vi "WILT Step 4.vi"(0 "Dryer Step 4 In":T8 {"Night Cycle Count" format="%04d"; "Day Cycle Count" format="%04d"}, 1 "Day/Night Cycle":T2, 2 "Step 3 Input":T6, 5 "Error In":errorcluster, 6 "Valve Status":T4, 7 "Agilent Valve and Switch Locations":T3[](array[typedef])=[{"Channel"="301", "Station"="1", "Label"="Water Valve", "Agilent Station"="2", "Data"=0.0}, {"Channel"="302", "Station"="2", "Label"="Water Valve", "Agilent Station"="2", "Data"=0.0}, {"Channel"="303", "Station"="3", "Label"="Water Valve", "Agilent Station"="2", "Data"=0.0}, {"Channel"="304", "Station"="4", "Label"="Water Valve", "Agilent Station"="2", "Data"=0.0}, {"Channel"="305", "Station"="5", "Label"="Water Valve", "Agilent Station"="2", "Data"=0.0}, {"Channel"="306", "Station"="6", "Label"="Water Valve", "Agilent Station"="2", "Data"=0.0}, {"Channel"="307", "Station"="7", "Label"="Water Valve", "Agilent Station"="2", "Data"=0.0}, {"Channel"="308", "Station"="8", "Label"="Water Valve", "Agilent Station"="2", "Data"=0.0}, {"Channel"="309", "Station"="9", "Label"="Water Valve", "Agilent Station"="2", "Data"=0.0}, {"Channel"="310", "Station"="10", "Label"="Water Valve", "Agilent Station"="2", "Data"=0.0}, {"Channel"="311", "Station"="11", "Label"="Water Valve", "Agilent Station"="2", "Data"=0.0}, {"Channel"="312", "Station"="12", "Label"="Water Valve", "Agilent Station"="2", "Data"=0.0}, {"Channel"="313", "Station"="13", "Label"="Water Valve", "Agilent Station"="2", "Data"=0.0}, {"Channel"="314", "Station"="14", "Label"="Water Valve", "Agilent Station"="2", "Data"=0.0}, {"Channel"="315", "Station"="15", "Label"="Water Valve", "Agilent Station"="2", "Data"=0.0}, {"Channel"="316", "Station"="16", "Label"="Water Valve", "Agilent Station"="2", "Data"=0.0}, {"Channel"="317", "Station"="17", "Label"="Water Valve", "Agilent Station"="2", "Data"=0.0}, {"Channel"="318", "Station"="18", "Label"="Water Valve", "Agilent Station"="2", "Data"=0.0}, {"Channel"="319", "Station"="19", "Label"="Water Valve", "Agilent Station"="2", "Data"=0.0}, {"Channel"="320", "Station"="20", "Label"="Water Valve", "Agilent Station"="2", "Data"=0.0}, {"Channel"="101", "Station"="21", "Label"="Water Valve", "Agilent Station"="3", "Data"=0.0}, {"Channel"="102", "Station"="22", "Label"="Water Valve", "Agilent Station"="3", "Data"=0.0}, {"Channel"="103", "Station"="23", "Label"="Water Valve", "Agilent Station"="3", "Data"=0.0}, {"Channel"="104", "Station"="24", "Label"="Water Valve", "Agilent Station"="3", "Data"=0.0}, {"Channel"="105", "Station"="25", "Label"="Water Valve", "Agilent Station"="3", "Data"=0.0}, {"Channel"="106", "Station"="26", "Label"="Water Valve", "Agilent Station"="3", "Data"=0.0}, {"Channel"="107", "Station"="27", "Label"="Water Valve", "Agilent Station"="3", "Data"=0.0}, {"Channel"="108", "Station"="28", "Label"="Water Valve", "Agilent Station"="3", "Data"=0.0}, {"Channel"="109", "Station"="29", "Label"="Water Valve", "Agilent Station"="3", "Data"=0.0}, {"Channel"="110", "Station"="30", "Label"="Water Valve", "Agilent Station"="3", "Data"=0.0}, {"Channel"="111", "Station"="31", "Label"="Water Valve", "Agilent Station"="3", "Data"=0.0}, {"Channel"="112", "Station"="32", "Label"="Water Valve", "Agilent Station"="3", "Data"=0.0}, {"Channel"="101", "Station"="33", "Label"="Water Valve", "Agilent Station"="5", "Data"=0.0}, {"Channel"="102", "Station"="34", "Label"="Water Valve", "Agilent Station"="5", "Data"=0.0}, {"Channel"="103", "Station"="35", "Label"="Water Valve", "Agilent Station"="5", "Data"=0.0}, {"Channel"="104", "Station"="36", "Label"="Water Valve", "Agilent Station"="5", "Data"=0.0}, {"Channel"="105", "Station"="37", "Label"="Water Valve", "Agilent Station"="5", "Data"=0.0}, {"Channel"="106", "Station"="38", "Label"="Water Valve", "Agilent Station"="5", "Data"=0.0}, {"Channel"="107", "Station"="39", "Label"="Water Valve", "Agilent Station"="5", "Data"=0.0}, {"Channel"="108", "Station"="40", "Label"="Water Valve", "Agilent Station"="5", "Data"=0.0}, {"Channel"="109", "Station"="41", "Label"="Water Valve", "Agilent Station"="5", "Data"=0.0}, {"Channel"="110", "Station"="42", "Label"="Water Valve", "Agilent Station"="5", "Data"=0.0}, {"Channel"="111", "Station"="43", "Label"="Water Valve", "Agilent Station"="5", "Data"=0.0}, {"Channel"="112", "Station"="44", "Label"="Water Valve", "Agilent Station"="5", "Data"=0.0}, {"Channel"="113", "Station"="45", "Label"="Water Valve", "Agilent Station"="5", "Data"=0.0}, {"Channel"="114", "Station"="46", "Label"="Water Valve", "Agilent Station"="5", "Data"=0.0}, {"Channel"="115", "Station"="47", "Label"="Water Valve", "Agilent Station"="5", "Data"=0.0}, {"Channel"="116", "Station"="48", "Label"="Water Valve", "Agilent Station"="5", "Data"=0.0}, {"Channel"="117", "Station"="49", "Label"="Water Valve", "Agilent Station"="5", "Data"=0.0}, {"Channel"="118", "Station"="50", "Label"="Water Valve", "Agilent Station"="5", "Data"=0.0}, {"Channel"="119", "Station"="51", "Label"="Water Valve", "Agilent Station"="5", "Data"=0.0}, {"Channel"="120", "Station"="52", "Label"="Water Valve", "Agilent Station"="5", "Data"=0.0}, {"Channel"="201", "Station"="53", "Label"="Water Valve", "Agilent Station"="5", "Data"=0.0}, {"Channel"="202", "Station"="54", "Label"="Water Valve", "Agilent Station"="5", "Data"=0.0}, {"Channel"="203", "Station"="55", "Label"="Water Valve", "Agilent Station"="5", "Data"=0.0}, {"Channel"="204", "Station"="56", "Label"="Water Valve", "Agilent Station"="5", "Data"=0.0}, {"Channel"="301", "Station"="21", "Label"="Start Button", "Agilent Station"="5", "Data"=0.0}, {"Channel"="302", "Station"="22", "Label"="Start Button", "Agilent Station"="5", "Data"=0.0}, {"Channel"="303", "Station"="23", "Label"="Start Button", "Agilent Station"="5", "Data"=0.0}, {"Channel"="304", "Station"="24", "Label"="Start Button", "Agilent Station"="5", "Data"=0.0}, {"Channel"="305", "Station"="25", "Label"="Start Button", "Agilent Station"="5", "Data"=0.0}, {"Channel"="306", "Station"="26", "Label"="Start Button", "Agilent Station"="5", "Data"=0.0}, {"Channel"="307", "Station"="27", "Label"="Start Button", "Agilent Station"="5", "Data"=0.0}, {"Channel"="308", "Station"="28", "Label"="Start Button", "Agilent Station"="5", "Data"=0.0}, {"Channel"="309", "Station"="29", "Label"="Start Button", "Agilent Station"="5", "Data"=0.0}, {"Channel"="310", "Station"="30", "Label"="Start Button", "Agilent Station"="5", "Data"=0.0}, {"Channel"="311", "Station"="31", "Label"="Start Button", "Agilent Station"="5", "Data"=0.0}, {"Channel"="312", "Station"="32", "Label"="Start Button", "Agilent Station"="5", "Data"=0.0}, {"Channel"="101", "Station"="33", "Label"="Start Button", "Agilent Station"="7", "Data"=0.0}, {"Channel"="102", "Station"="34", "Label"="Start Button", "Agilent Station"="7", "Data"=0.0}, {"Channel"="103", "Station"="35", "Label"="Start Button", "Agilent Station"="7", "Data"=0.0}, {"Channel"="104", "Station"="36", "Label"="Start Button", "Agilent Station"="7", "Data"=0.0}, {"Channel"="105", "Station"="37", "Label"="Start Button", "Agilent Station"="7", "Data"=0.0}, {"Channel"="106", "Station"="38", "Label"="Start Button", "Agilent Station"="7", "Data"=0.0}, {"Channel"="107", "Station"="39", "Label"="Start Button", "Agilent Station"="7", "Data"=0.0}, {"Channel"="108", "Station"="40", "Label"="Start Button", "Agilent Station"="7", "Data"=0.0}, {"Channel"="109", "Station"="41", "Label"="Start Button", "Agilent Station"="7", "Data"=0.0}, {"Channel"="110", "Station"="42", "Label"="Start Button", "Agilent Station"="7", "Data"=0.0}, {"Channel"="111", "Station"="43", "Label"="Start Button", "Agilent Station"="7", "Data"=0.0}, {"Channel"="112", "Station"="44", "Label"="Start Button", "Agilent Station"="7", "Data"=0.0}, {"Channel"="113", "Station"="45", "Label"="Start Button", "Agilent Station"="7", "Data"=0.0}, {"Channel"="114", "Station"="46", "Label"="Start Button", "Agilent Station"="7", "Data"=0.0}, {"Channel"="115", "Station"="47", "Label"="Start Button", "Agilent Station"="7", "Data"=0.0}, {"Channel"="116", "Station"="48", "Label"="Start Button", "Agilent Station"="7", "Data"=0.0}, {"Channel"="117", "Station"="49", "Label"="Start Button", "Agilent Station"="7", "Data"=0.0}, {"Channel"="118", "Station"="50", "Label"="Start Button", "Agilent Station"="7", "Data"=0.0}, {"Channel"="119", "Station"="51", "Label"="Start Button", "Agilent Station"="7", "Data"=0.0}, {"Channel"="120", "Station"="52", "Label"="Start Button", "Agilent Station"="7", "Data"=0.0}, {"Channel"="201", "Station"="53", "Label"="Start Button", "Agilent Station"="7", "Data"=0.0}, {"Channel"="202", "Station"="54", "Label"="Start Button", "Agilent Station"="7", "Data"=0.0}, {"Channel"="203", "Station"="55", "Label"="Start Button", "Agilent Station"="7", "Data"=0.0}, {"Channel"="204", "Station"="56", "Label"="Start Button", "Agilent Station"="7", "Data"=0.0}], 8 "Station Number in":u32, 10 "Station Group":T5, 11 "Semaphore":T1[](array[typedef])) -> (14 "Dryer Step 4 Output":T8 {"Night Cycle Count" format="%04d"; "Day Cycle Count" format="%04d"}, 16 "Step 3 Output":T6, 19 "Error Out":errorcluster)   [LabVIEW 2016]
uses:
  Type Definitions/WILT Station Test State Cluster.ctl
  Type Definitions/WILT Dryer Test State.ctl
  Type Definitions/WILT Dryer.ctl
  Type Definitions/WILT Dryer Details.ctl
  Type Definitions/WILT Agilent Channel Definition.ctl
  Type Definitions/WILT DAQ Data.ctl
  Type Definitions/WILT Room Location.ctl
  Type Definitions/WILT Water Valve Control.ctl
  Type Definitions/WILT Day Night Cycle Enum.ctl
  Globals/WILT Globals Main Program.vi
panel:
  # "Day"
  # "Night"
  # "Day"
  # "Night"
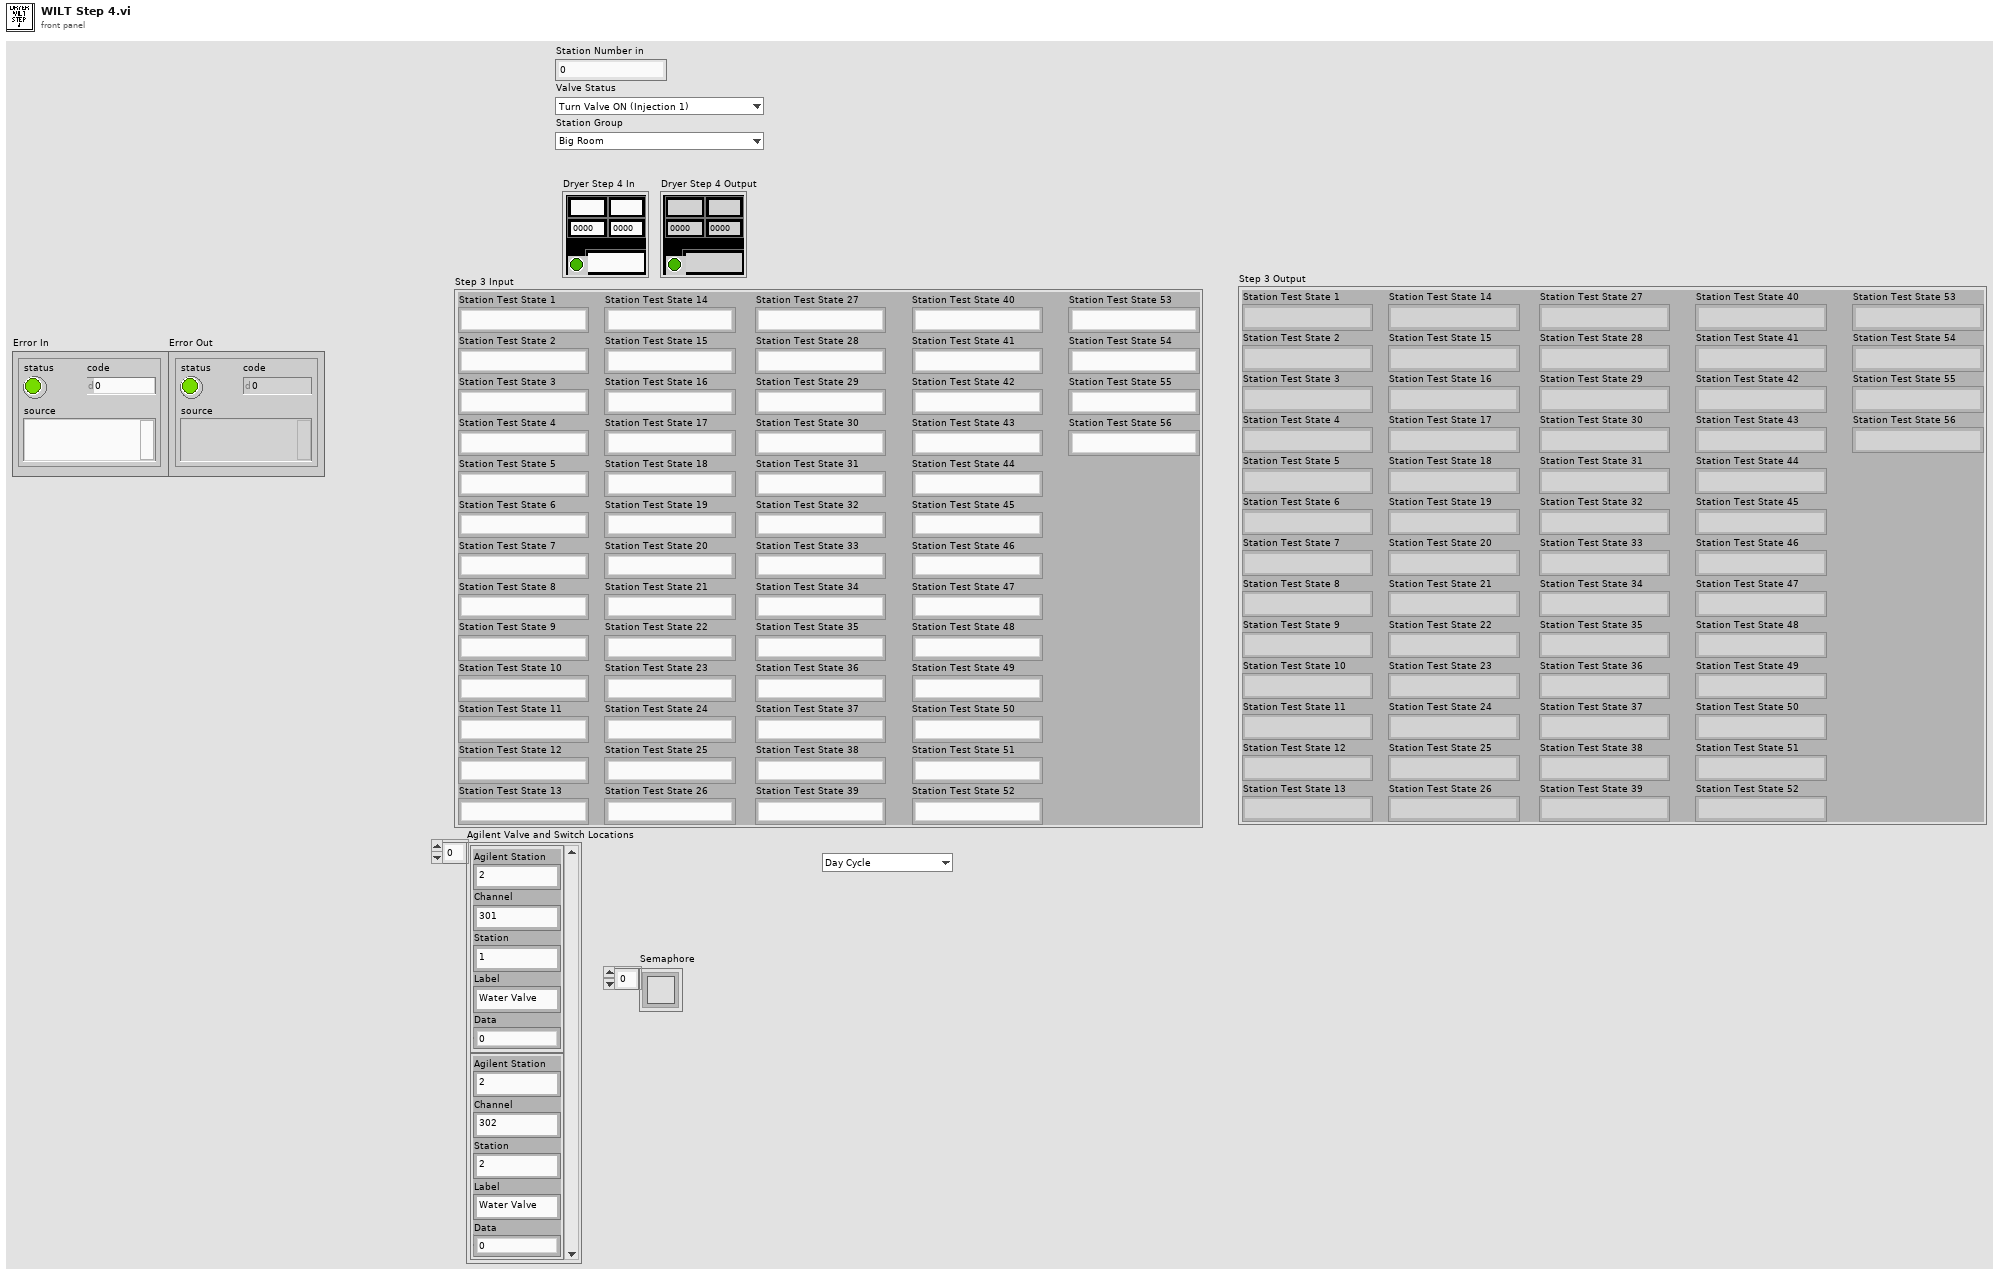
[diagram p1: front panel]
types:
  T1 = typedef "Semaphore RefNum" = refnum<k1>
  T2 = typedef "WILT Day Night Cycle Enum.ctl" = enum16{"Day Cycle", "Night Cycle", "Day Cycle (No Water)"}
  T3 = typedef "WILT Agilent Channel Definition.ctl" = cluster{"Channel":string, "Station":string, "Label":string, "Agilent Station":string, "Data":dbl}
  T4 = typedef "WILT Water Valve Control.ctl" = enum16{"Turn Valve ON (Injection 1)", "Turn Valve OFF (Injection 1)", "Turn Valve ON (Injection 2)", "Turn Valve OFF (Injection 2)"}
  T5 = typedef "WILT Room Location.ctl" = enum16{"Big Room", "Remote Stations"}
  T6 = typedef "WILT Station Test State Cluster.ctl" = cluster{"Station Test State 1":T7, "Station Test State 2":T7, "Station Test State 3":T7, "Station Test State 4":T7, "Station Test State 5":T7, "Station Test State 6":T7, "Station Test State 7":T7, "Station Test State 8":T7, "Station Test State 9":T7, "Station Test State 10":T7, "Station Test State 11":T7, "Station Test State 12":T7, "Station Test State 13":T7, "Station Test State 14":T7, "Station Test State 15":T7, "Station Test State 16":T7, "Station Test State 17":T7, "Station Test State 18":T7, "Station Test State 19":T7, "Station Test State 20":T7, "Station Test State 21":T7, "Station Test State 22":T7, "Station Test State 23":T7, "Station Test State 24":T7, "Station Test State 25":T7, "Station Test State 26":T7, "Station Test State 27":T7, "Station Test State 28":T7, "Station Test State 29":T7, "Station Test State 30":T7, "Station Test State 31":T7, "Station Test State 32":T7, "Station Test State 33":T7, "Station Test State 34":T7, "Station Test State 35":T7, "Station Test State 36":T7, "Station Test State 37":T7, "Station Test State 38":T7, "Station Test State 39":T7, "Station Test State 40":T7, "Station Test State 41":T7, "Station Test State 42":T7, "Station Test State 43":T7, "Station Test State 44":T7, "Station Test State 45":T7, "Station Test State 46":T7, "Station Test State 47":T7, "Station Test State 48":T7, "Station Test State 49":T7, "Station Test State 50":T7, "Station Test State 51":T7, "Station Test State 52":T7, "Station Test State 53":T7, "Station Test State 54":T7, "Station Test State 55":T7, "Station Test State 56":T7}
  T7 = typedef "WILT Dryer Test State.ctl" = enum16{"No Serial Number", "Waiting for Dryer To Start", "Drying Clothes", "Water Injection 1 (On)", "Water Injection 1 Timer", "Water Injection 1 (Off)", "Pause Dryer", "Sending Start Stop CMD", "Pause Dryer 2", "Sending Start Stop CMD 2", "Drying Clothes 2", "Water Injection 2 (On)", "Water Injection 2 Timer", "Water Injection 2 (Off)", "Drying Clothes 3", "Cooling Down", "Sending Start Stop CMD 3", "Increment Cycle"}
  T8 = typedef "WILT Dryer.ctl" = cluster{"Lab ID":string, "Day Cycle Count":i32, "Station Label":string, "Dryer Details":T9, "Status Color":u32, "Invisible Button":bool, "Night Cycle Count":i32, "Station Index":i32, "Cycle Index":string, "Audit Alert":bool, "Agilent Channel Definition":T3, "DAQ Data":T10}
  T9 = typedef "WILT Dryer Details.ctl" = cluster{"Station":string, "Lab ID":string, "TR Number":string}
  T10 = typedef "WILT DAQ Data.ctl" = cluster{"L1 Current":dbl, "L2 Current":dbl, "Temperature  Deg F (TC)":dbl, "Volts":dbl, "Volts (208)":dbl, "SW (208)":dbl}
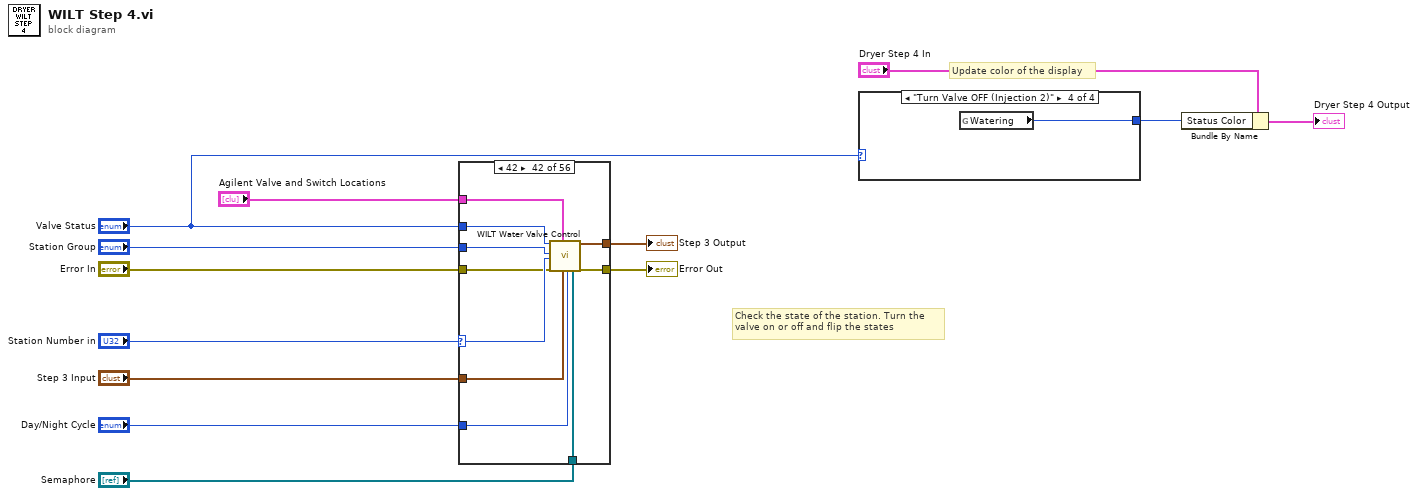
[diagram p0: block diagram]
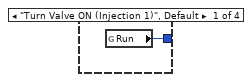
[diagram p2: hidden frame]
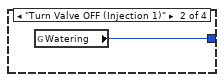
[diagram p3: hidden frame]
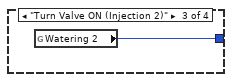
[diagram p4: hidden frame]
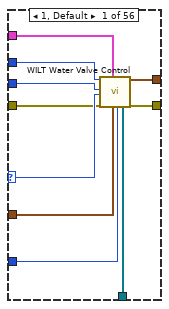
[diagram p5: hidden frame]
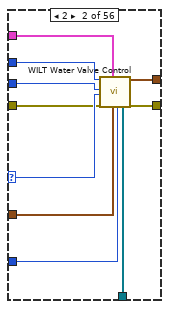
[diagram p6: hidden frame]
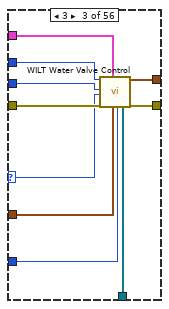
[diagram p7: hidden frame]
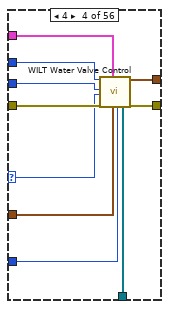
[diagram p8: hidden frame]
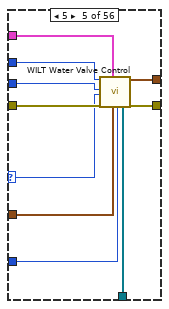
[diagram p9: hidden frame]
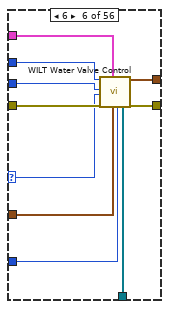
[diagram p10: hidden frame]
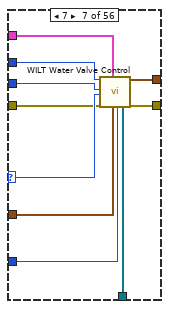
[diagram p11: hidden frame]
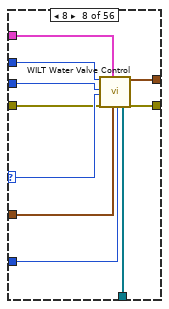
[diagram p12: hidden frame]
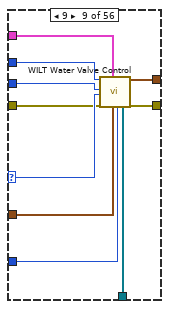
[diagram p13: hidden frame]
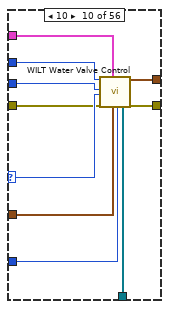
[diagram p14: hidden frame]
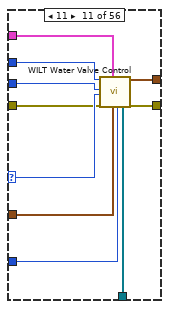
[diagram p15: hidden frame]
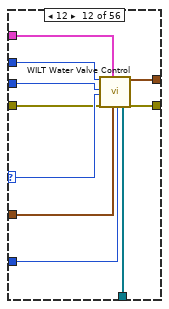
[diagram p16: hidden frame]
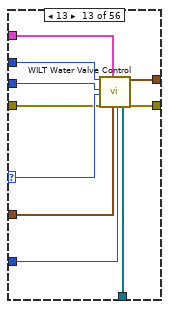
[diagram p17: hidden frame]
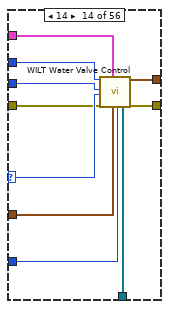
[diagram p18: hidden frame]
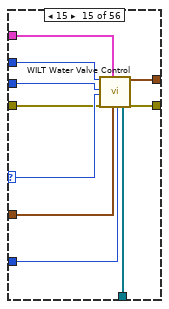
[diagram p19: hidden frame]
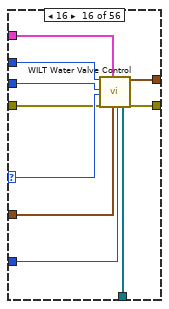
[diagram p20: hidden frame]
diagram:
  # "Update color of the display"
  # "Check the state of the station. Turn the \nvalve on or off and flip the states"
  n1 = case shown="42" "Station Number in" {
    selector: "Station Number in" -> [w21 w31 w38 w50 w58 w68 w81 w91 w101 w111 w121 w131 w141 w151 w161 w171 w181 w191 w201 w211 w221 w231 w241 w251 w261 w271 w281 w291 w301 w311 w321 w331 w341 w351 w361 w371 w381 w391 w401 w411 w421 w431 w441 w451 w461 w471 w481 w490 w501 w511 w521 w531 w541 w551 w561 w572]
    tunnel: "Step 3 Input" -> [w19 w29 w39 w51 w61 w71 w80 w89 w99 w109 w120 w130 w139 w149 w159 w169 w179 w189 w199 w209 w219 w230 w239 w249 w259 w269 w279 w289 w299 w309 w319 w329 w339 w349 w359 w369 w379 w389 w399 w409 w419 w430 w440 w449 w459 w469 w479 w493 w499 w509 w519 w529 w539 w549 w559 w571]
    tunnel: "Valve Status" -> [w23 w33 w43 w48 w59 w69 w83 w93 w103 w113 w123 w133 w143 w153 w163 w173 w183 w193 w203 w213 w223 w233 w243 w253 w263 w273 w283 w293 w303 w313 w323 w333 w343 w353 w363 w373 w383 w393 w403 w413 w423 w433 w443 w453 w463 w473 w483 w492 w503 w513 w523 w533 w543 w552 w563 w569]
    tunnel: "Station Group" -> [w22 w32 w37 w49 w60 w70 w82 w92 w102 w112 w122 w132 w142 w152 w162 w172 w182 w192 w202 w212 w222 w232 w242 w252 w262 w272 w282 w292 w302 w312 w322 w332 w342 w352 w362 w372 w382 w392 w402 w412 w422 w432 w442 w452 w462 w472 w482 w491 w502 w512 w522 w532 w542 w553 w562 w573]
    tunnel: [w18 w28 w42 w47 w57 w67 w77 w88 w98 w108 w117 w127 w138 w148 w158 w168 w178 w188 w198 w208 w218 w228 w238 w248 w258 w268 w278 w288 w298 w308 w318 w328 w338 w348 w358 w368 w378 w388 w398 w408 w418 w428 w438 w448 w458 w468 w478 w487 w498 w508 w518 w528 w538 w548 w558 w570] -> w7
    tunnel: "Error In" -> [w20 w30 w40 w53 w63 w73 w79 w90 w100 w110 w119 w129 w140 w150 w160 w170 w180 w190 w200 w210 w220 w229 w240 w250 w260 w270 w280 w290 w300 w310 w320 w330 w340 w350 w360 w370 w380 w390 w400 w410 w420 w429 w439 w450 w460 w470 w480 w489 w500 w510 w520 w530 w540 w550 w560 w568]
    tunnel: [w17 w27 w41 w52 w62 w72 w78 w87 w97 w107 w118 w128 w137 w147 w157 w167 w177 w187 w197 w207 w217 w227 w237 w247 w257 w267 w277 w287 w297 w307 w317 w327 w337 w347 w357 w367 w377 w387 w397 w407 w417 w427 w437 w447 w457 w467 w477 w488 w497 w507 w517 w527 w537 w547 w557 w567] -> w6
    tunnel: "Agilent Valve and Switch Locations" -> [w16 w26 w36 w46 w56 w66 w76 w86 w96 w106 w116 w126 w136 w146 w156 w166 w176 w186 w196 w206 w216 w226 w236 w246 w256 w266 w276 w286 w296 w306 w316 w326 w336 w346 w356 w366 w376 w386 w396 w406 w416 w426 w436 w446 w456 w466 w476 w486 w496 w506 w516 w526 w536 w546 w556 w566]
    tunnel: "Day/Night Cycle" -> [w15 w25 w35 w45 w55 w65 w75 w85 w95 w105 w115 w125 w135 w145 w155 w165 w175 w185 w195 w205 w215 w225 w235 w245 w255 w265 w275 w285 w295 w305 w315 w325 w335 w345 w355 w365 w375 w385 w395 w405 w415 w425 w435 w445 w455 w465 w475 w485 w495 w505 w515 w525 w535 w545 w555 w565]
    tunnel: "Semaphore" -> [w14 w24 w34 w44 w54 w64 w74 w84 w94 w104 w114 w124 w134 w144 w154 w164 w174 w184 w194 w204 w214 w224 w234 w244 w254 w264 w274 w284 w294 w304 w314 w324 w334 w344 w354 w364 w374 w384 w394 w404 w414 w424 w434 w444 w454 w464 w474 w484 w494 w504 w514 w524 w534 w544 w554 w564]
    frame 1, Default {
      n2 = call "WILT Water Valve Control.vi"("Valve Status"=w23, "Station Group"=w22, "Station Number"=w21, "Error In"=w20, "Agilent Valve and Switch Locations"=w16, "Step 3 Input in"=w19, "Day/Night Cycle"=w15, "Semaphore"=w14) -> ("Step 3 Input out"=w18:T6, "Error Out"=w17:errorcluster)  [unwired: 10 in]
    }
    frame 2 {
      n3 = call "WILT Water Valve Control.vi"("Valve Status"=w33, "Station Group"=w32, "Station Number"=w31, "Error In"=w30, "Agilent Valve and Switch Locations"=w26, "Step 3 Input in"=w29, "Day/Night Cycle"=w25, "Semaphore"=w24) -> ("Step 3 Input out"=w28:T6, "Error Out"=w27:errorcluster)  [unwired: 10 in]
    }
    frame 3 {
      n4 = call "WILT Water Valve Control.vi"("Valve Status"=w43, "Station Group"=w37, "Station Number"=w38, "Error In"=w40, "Agilent Valve and Switch Locations"=w36, "Step 3 Input in"=w39, "Day/Night Cycle"=w35, "Semaphore"=w34) -> ("Step 3 Input out"=w42:T6, "Error Out"=w41:errorcluster)  [unwired: 10 in]
    }
    frame 4 {
      n5 = call "WILT Water Valve Control.vi"("Valve Status"=w48, "Station Group"=w49, "Station Number"=w50, "Error In"=w53, "Agilent Valve and Switch Locations"=w46, "Step 3 Input in"=w51, "Day/Night Cycle"=w45, "Semaphore"=w44) -> ("Step 3 Input out"=w47:T6, "Error Out"=w52:errorcluster)  [unwired: 10 in]
    }
    frame 5 {
      n6 = call "WILT Water Valve Control.vi"("Valve Status"=w59, "Station Group"=w60, "Station Number"=w58, "Error In"=w63, "Agilent Valve and Switch Locations"=w56, "Step 3 Input in"=w61, "Day/Night Cycle"=w55, "Semaphore"=w54) -> ("Step 3 Input out"=w57:T6, "Error Out"=w62:errorcluster)  [unwired: 10 in]
    }
    frame 6 {
      n7 = call "WILT Water Valve Control.vi"("Valve Status"=w69, "Station Group"=w70, "Station Number"=w68, "Error In"=w73, "Agilent Valve and Switch Locations"=w66, "Step 3 Input in"=w71, "Day/Night Cycle"=w65, "Semaphore"=w64) -> ("Step 3 Input out"=w67:T6, "Error Out"=w72:errorcluster)  [unwired: 10 in]
    }
    frame 7 {
      n8 = call "WILT Water Valve Control.vi"("Valve Status"=w83, "Station Group"=w82, "Station Number"=w81, "Error In"=w79, "Agilent Valve and Switch Locations"=w76, "Step 3 Input in"=w80, "Day/Night Cycle"=w75, "Semaphore"=w74) -> ("Step 3 Input out"=w77:T6, "Error Out"=w78:errorcluster)  [unwired: 10 in]
    }
    frame 8 {
      n9 = call "WILT Water Valve Control.vi"("Valve Status"=w93, "Station Group"=w92, "Station Number"=w91, "Error In"=w90, "Agilent Valve and Switch Locations"=w86, "Step 3 Input in"=w89, "Day/Night Cycle"=w85, "Semaphore"=w84) -> ("Step 3 Input out"=w88:T6, "Error Out"=w87:errorcluster)  [unwired: 10 in]
    }
    frame 9 {
      n10 = call "WILT Water Valve Control.vi"("Valve Status"=w103, "Station Group"=w102, "Station Number"=w101, "Error In"=w100, "Agilent Valve and Switch Locations"=w96, "Step 3 Input in"=w99, "Day/Night Cycle"=w95, "Semaphore"=w94) -> ("Step 3 Input out"=w98:T6, "Error Out"=w97:errorcluster)  [unwired: 10 in]
    }
    frame 10 {
      n11 = call "WILT Water Valve Control.vi"("Valve Status"=w113, "Station Group"=w112, "Station Number"=w111, "Error In"=w110, "Agilent Valve and Switch Locations"=w106, "Step 3 Input in"=w109, "Day/Night Cycle"=w105, "Semaphore"=w104) -> ("Step 3 Input out"=w108:T6, "Error Out"=w107:errorcluster)  [unwired: 10 in]
    }
    frame 11 {
      n12 = call "WILT Water Valve Control.vi"("Valve Status"=w123, "Station Group"=w122, "Station Number"=w121, "Error In"=w119, "Agilent Valve and Switch Locations"=w116, "Step 3 Input in"=w120, "Day/Night Cycle"=w115, "Semaphore"=w114) -> ("Step 3 Input out"=w117:T6, "Error Out"=w118:errorcluster)  [unwired: 10 in]
    }
    frame 12 {
      n13 = call "WILT Water Valve Control.vi"("Valve Status"=w133, "Station Group"=w132, "Station Number"=w131, "Error In"=w129, "Agilent Valve and Switch Locations"=w126, "Step 3 Input in"=w130, "Day/Night Cycle"=w125, "Semaphore"=w124) -> ("Step 3 Input out"=w127:T6, "Error Out"=w128:errorcluster)  [unwired: 10 in]
    }
    frame 13 {
      n14 = call "WILT Water Valve Control.vi"("Valve Status"=w143, "Station Group"=w142, "Station Number"=w141, "Error In"=w140, "Agilent Valve and Switch Locations"=w136, "Step 3 Input in"=w139, "Day/Night Cycle"=w135, "Semaphore"=w134) -> ("Step 3 Input out"=w138:T6, "Error Out"=w137:errorcluster)  [unwired: 10 in]
    }
    frame 14 {
      n15 = call "WILT Water Valve Control.vi"("Valve Status"=w153, "Station Group"=w152, "Station Number"=w151, "Error In"=w150, "Agilent Valve and Switch Locations"=w146, "Step 3 Input in"=w149, "Day/Night Cycle"=w145, "Semaphore"=w144) -> ("Step 3 Input out"=w148:T6, "Error Out"=w147:errorcluster)  [unwired: 10 in]
    }
    frame 15 {
      n16 = call "WILT Water Valve Control.vi"("Valve Status"=w163, "Station Group"=w162, "Station Number"=w161, "Error In"=w160, "Agilent Valve and Switch Locations"=w156, "Step 3 Input in"=w159, "Day/Night Cycle"=w155, "Semaphore"=w154) -> ("Step 3 Input out"=w158:T6, "Error Out"=w157:errorcluster)  [unwired: 10 in]
    }
    frame 16 {
      n17 = call "WILT Water Valve Control.vi"("Valve Status"=w173, "Station Group"=w172, "Station Number"=w171, "Error In"=w170, "Agilent Valve and Switch Locations"=w166, "Step 3 Input in"=w169, "Day/Night Cycle"=w165, "Semaphore"=w164) -> ("Step 3 Input out"=w168:T6, "Error Out"=w167:errorcluster)  [unwired: 10 in]
    }
    frame 17 {
      n18 = call "WILT Water Valve Control.vi"("Valve Status"=w183, "Station Group"=w182, "Station Number"=w181, "Error In"=w180, "Agilent Valve and Switch Locations"=w176, "Step 3 Input in"=w179, "Day/Night Cycle"=w175, "Semaphore"=w174) -> ("Step 3 Input out"=w178:T6, "Error Out"=w177:errorcluster)  [unwired: 10 in]
    }
    frame 18 {
      n19 = call "WILT Water Valve Control.vi"("Valve Status"=w193, "Station Group"=w192, "Station Number"=w191, "Error In"=w190, "Agilent Valve and Switch Locations"=w186, "Step 3 Input in"=w189, "Day/Night Cycle"=w185, "Semaphore"=w184) -> ("Step 3 Input out"=w188:T6, "Error Out"=w187:errorcluster)  [unwired: 10 in]
    }
    frame 19 {
      n20 = call "WILT Water Valve Control.vi"("Valve Status"=w203, "Station Group"=w202, "Station Number"=w201, "Error In"=w200, "Agilent Valve and Switch Locations"=w196, "Step 3 Input in"=w199, "Day/Night Cycle"=w195, "Semaphore"=w194) -> ("Step 3 Input out"=w198:T6, "Error Out"=w197:errorcluster)  [unwired: 10 in]
    }
    frame 20 {
      n21 = call "WILT Water Valve Control.vi"("Valve Status"=w213, "Station Group"=w212, "Station Number"=w211, "Error In"=w210, "Agilent Valve and Switch Locations"=w206, "Step 3 Input in"=w209, "Day/Night Cycle"=w205, "Semaphore"=w204) -> ("Step 3 Input out"=w208:T6, "Error Out"=w207:errorcluster)  [unwired: 10 in]
    }
    frame 21 {
      n22 = call "WILT Water Valve Control.vi"("Valve Status"=w223, "Station Group"=w222, "Station Number"=w221, "Error In"=w220, "Agilent Valve and Switch Locations"=w216, "Step 3 Input in"=w219, "Day/Night Cycle"=w215, "Semaphore"=w214) -> ("Step 3 Input out"=w218:T6, "Error Out"=w217:errorcluster)  [unwired: 10 in]
    }
    frame 22 {
      n23 = call "WILT Water Valve Control.vi"("Valve Status"=w233, "Station Group"=w232, "Station Number"=w231, "Error In"=w229, "Agilent Valve and Switch Locations"=w226, "Step 3 Input in"=w230, "Day/Night Cycle"=w225, "Semaphore"=w224) -> ("Step 3 Input out"=w228:T6, "Error Out"=w227:errorcluster)  [unwired: 10 in]
    }
    frame 23 {
      n24 = call "WILT Water Valve Control.vi"("Valve Status"=w243, "Station Group"=w242, "Station Number"=w241, "Error In"=w240, "Agilent Valve and Switch Locations"=w236, "Step 3 Input in"=w239, "Day/Night Cycle"=w235, "Semaphore"=w234) -> ("Step 3 Input out"=w238:T6, "Error Out"=w237:errorcluster)  [unwired: 10 in]
    }
    frame 24 {
      n25 = call "WILT Water Valve Control.vi"("Valve Status"=w253, "Station Group"=w252, "Station Number"=w251, "Error In"=w250, "Agilent Valve and Switch Locations"=w246, "Step 3 Input in"=w249, "Day/Night Cycle"=w245, "Semaphore"=w244) -> ("Step 3 Input out"=w248:T6, "Error Out"=w247:errorcluster)  [unwired: 10 in]
    }
    frame 25 {
      n26 = call "WILT Water Valve Control.vi"("Valve Status"=w263, "Station Group"=w262, "Station Number"=w261, "Error In"=w260, "Agilent Valve and Switch Locations"=w256, "Step 3 Input in"=w259, "Day/Night Cycle"=w255, "Semaphore"=w254) -> ("Step 3 Input out"=w258:T6, "Error Out"=w257:errorcluster)  [unwired: 10 in]
    }
    frame 26 {
      n27 = call "WILT Water Valve Control.vi"("Valve Status"=w273, "Station Group"=w272, "Station Number"=w271, "Error In"=w270, "Agilent Valve and Switch Locations"=w266, "Step 3 Input in"=w269, "Day/Night Cycle"=w265, "Semaphore"=w264) -> ("Step 3 Input out"=w268:T6, "Error Out"=w267:errorcluster)  [unwired: 10 in]
    }
    frame 27 {
      n28 = call "WILT Water Valve Control.vi"("Valve Status"=w283, "Station Group"=w282, "Station Number"=w281, "Error In"=w280, "Agilent Valve and Switch Locations"=w276, "Step 3 Input in"=w279, "Day/Night Cycle"=w275, "Semaphore"=w274) -> ("Step 3 Input out"=w278:T6, "Error Out"=w277:errorcluster)  [unwired: 10 in]
    }
    frame 28 {
      n29 = call "WILT Water Valve Control.vi"("Valve Status"=w293, "Station Group"=w292, "Station Number"=w291, "Error In"=w290, "Agilent Valve and Switch Locations"=w286, "Step 3 Input in"=w289, "Day/Night Cycle"=w285, "Semaphore"=w284) -> ("Step 3 Input out"=w288:T6, "Error Out"=w287:errorcluster)  [unwired: 10 in]
    }
    frame 29 {
      n30 = call "WILT Water Valve Control.vi"("Valve Status"=w303, "Station Group"=w302, "Station Number"=w301, "Error In"=w300, "Agilent Valve and Switch Locations"=w296, "Step 3 Input in"=w299, "Day/Night Cycle"=w295, "Semaphore"=w294) -> ("Step 3 Input out"=w298:T6, "Error Out"=w297:errorcluster)  [unwired: 10 in]
    }
    frame 30 {
      n31 = call "WILT Water Valve Control.vi"("Valve Status"=w313, "Station Group"=w312, "Station Number"=w311, "Error In"=w310, "Agilent Valve and Switch Locations"=w306, "Step 3 Input in"=w309, "Day/Night Cycle"=w305, "Semaphore"=w304) -> ("Step 3 Input out"=w308:T6, "Error Out"=w307:errorcluster)  [unwired: 10 in]
    }
    frame 31 {
      n32 = call "WILT Water Valve Control.vi"("Valve Status"=w323, "Station Group"=w322, "Station Number"=w321, "Error In"=w320, "Agilent Valve and Switch Locations"=w316, "Step 3 Input in"=w319, "Day/Night Cycle"=w315, "Semaphore"=w314) -> ("Step 3 Input out"=w318:T6, "Error Out"=w317:errorcluster)  [unwired: 10 in]
    }
    frame 32 {
      n33 = call "WILT Water Valve Control.vi"("Valve Status"=w333, "Station Group"=w332, "Station Number"=w331, "Error In"=w330, "Agilent Valve and Switch Locations"=w326, "Step 3 Input in"=w329, "Day/Night Cycle"=w325, "Semaphore"=w324) -> ("Step 3 Input out"=w328:T6, "Error Out"=w327:errorcluster)  [unwired: 10 in]
    }
    frame 33 {
      n34 = call "WILT Water Valve Control.vi"("Valve Status"=w343, "Station Group"=w342, "Station Number"=w341, "Error In"=w340, "Agilent Valve and Switch Locations"=w336, "Step 3 Input in"=w339, "Day/Night Cycle"=w335, "Semaphore"=w334) -> ("Step 3 Input out"=w338:T6, "Error Out"=w337:errorcluster)  [unwired: 10 in]
    }
    frame 34 {
      n35 = call "WILT Water Valve Control.vi"("Valve Status"=w353, "Station Group"=w352, "Station Number"=w351, "Error In"=w350, "Agilent Valve and Switch Locations"=w346, "Step 3 Input in"=w349, "Day/Night Cycle"=w345, "Semaphore"=w344) -> ("Step 3 Input out"=w348:T6, "Error Out"=w347:errorcluster)  [unwired: 10 in]
    }
    frame 35 {
      n36 = call "WILT Water Valve Control.vi"("Valve Status"=w363, "Station Group"=w362, "Station Number"=w361, "Error In"=w360, "Agilent Valve and Switch Locations"=w356, "Step 3 Input in"=w359, "Day/Night Cycle"=w355, "Semaphore"=w354) -> ("Step 3 Input out"=w358:T6, "Error Out"=w357:errorcluster)  [unwired: 10 in]
    }
    frame 36 {
      n37 = call "WILT Water Valve Control.vi"("Valve Status"=w373, "Station Group"=w372, "Station Number"=w371, "Error In"=w370, "Agilent Valve and Switch Locations"=w366, "Step 3 Input in"=w369, "Day/Night Cycle"=w365, "Semaphore"=w364) -> ("Step 3 Input out"=w368:T6, "Error Out"=w367:errorcluster)  [unwired: 10 in]
    }
    frame 37 {
      n38 = call "WILT Water Valve Control.vi"("Valve Status"=w383, "Station Group"=w382, "Station Number"=w381, "Error In"=w380, "Agilent Valve and Switch Locations"=w376, "Step 3 Input in"=w379, "Day/Night Cycle"=w375, "Semaphore"=w374) -> ("Step 3 Input out"=w378:T6, "Error Out"=w377:errorcluster)  [unwired: 10 in]
    }
    frame 38 {
      n39 = call "WILT Water Valve Control.vi"("Valve Status"=w393, "Station Group"=w392, "Station Number"=w391, "Error In"=w390, "Agilent Valve and Switch Locations"=w386, "Step 3 Input in"=w389, "Day/Night Cycle"=w385, "Semaphore"=w384) -> ("Step 3 Input out"=w388:T6, "Error Out"=w387:errorcluster)  [unwired: 10 in]
    }
    frame 39 {
      n40 = call "WILT Water Valve Control.vi"("Valve Status"=w403, "Station Group"=w402, "Station Number"=w401, "Error In"=w400, "Agilent Valve and Switch Locations"=w396, "Step 3 Input in"=w399, "Day/Night Cycle"=w395, "Semaphore"=w394) -> ("Step 3 Input out"=w398:T6, "Error Out"=w397:errorcluster)  [unwired: 10 in]
    }
    frame 40 {
      n41 = call "WILT Water Valve Control.vi"("Valve Status"=w413, "Station Group"=w412, "Station Number"=w411, "Error In"=w410, "Agilent Valve and Switch Locations"=w406, "Step 3 Input in"=w409, "Day/Night Cycle"=w405, "Semaphore"=w404) -> ("Step 3 Input out"=w408:T6, "Error Out"=w407:errorcluster)  [unwired: 10 in]
    }
    frame 41 {
      n42 = call "WILT Water Valve Control.vi"("Valve Status"=w423, "Station Group"=w422, "Station Number"=w421, "Error In"=w420, "Agilent Valve and Switch Locations"=w416, "Step 3 Input in"=w419, "Day/Night Cycle"=w415, "Semaphore"=w414) -> ("Step 3 Input out"=w418:T6, "Error Out"=w417:errorcluster)  [unwired: 10 in]
    }
    frame 42 {
      n43 = call "WILT Water Valve Control.vi"("Valve Status"=w433, "Station Group"=w432, "Station Number"=w431, "Error In"=w429, "Agilent Valve and Switch Locations"=w426, "Step 3 Input in"=w430, "Day/Night Cycle"=w425, "Semaphore"=w424) -> ("Step 3 Input out"=w428:T6, "Error Out"=w427:errorcluster)  [unwired: 10 in]
    }
    frame 43 {
      n44 = call "WILT Water Valve Control.vi"("Valve Status"=w443, "Station Group"=w442, "Station Number"=w441, "Error In"=w439, "Agilent Valve and Switch Locations"=w436, "Step 3 Input in"=w440, "Day/Night Cycle"=w435, "Semaphore"=w434) -> ("Step 3 Input out"=w438:T6, "Error Out"=w437:errorcluster)  [unwired: 10 in]
    }
    frame 44 {
      n45 = call "WILT Water Valve Control.vi"("Valve Status"=w453, "Station Group"=w452, "Station Number"=w451, "Error In"=w450, "Agilent Valve and Switch Locations"=w446, "Step 3 Input in"=w449, "Day/Night Cycle"=w445, "Semaphore"=w444) -> ("Step 3 Input out"=w448:T6, "Error Out"=w447:errorcluster)  [unwired: 10 in]
    }
    frame 45 {
      n46 = call "WILT Water Valve Control.vi"("Valve Status"=w463, "Station Group"=w462, "Station Number"=w461, "Error In"=w460, "Agilent Valve and Switch Locations"=w456, "Step 3 Input in"=w459, "Day/Night Cycle"=w455, "Semaphore"=w454) -> ("Step 3 Input out"=w458:T6, "Error Out"=w457:errorcluster)  [unwired: 10 in]
    }
    frame 46 {
      n47 = call "WILT Water Valve Control.vi"("Valve Status"=w473, "Station Group"=w472, "Station Number"=w471, "Error In"=w470, "Agilent Valve and Switch Locations"=w466, "Step 3 Input in"=w469, "Day/Night Cycle"=w465, "Semaphore"=w464) -> ("Step 3 Input out"=w468:T6, "Error Out"=w467:errorcluster)  [unwired: 10 in]
    }
    frame 47 {
      n48 = call "WILT Water Valve Control.vi"("Valve Status"=w483, "Station Group"=w482, "Station Number"=w481, "Error In"=w480, "Agilent Valve and Switch Locations"=w476, "Step 3 Input in"=w479, "Day/Night Cycle"=w475, "Semaphore"=w474) -> ("Step 3 Input out"=w478:T6, "Error Out"=w477:errorcluster)  [unwired: 10 in]
    }
    frame 48 {
      n49 = call "WILT Water Valve Control.vi"("Valve Status"=w492, "Station Group"=w491, "Station Number"=w490, "Error In"=w489, "Agilent Valve and Switch Locations"=w486, "Step 3 Input in"=w493, "Day/Night Cycle"=w485, "Semaphore"=w484) -> ("Step 3 Input out"=w487:T6, "Error Out"=w488:errorcluster)  [unwired: 10 in]
    }
    frame 49 {
      n50 = call "WILT Water Valve Control.vi"("Valve Status"=w503, "Station Group"=w502, "Station Number"=w501, "Error In"=w500, "Agilent Valve and Switch Locations"=w496, "Step 3 Input in"=w499, "Day/Night Cycle"=w495, "Semaphore"=w494) -> ("Step 3 Input out"=w498:T6, "Error Out"=w497:errorcluster)  [unwired: 10 in]
    }
    frame 50 {
      n51 = call "WILT Water Valve Control.vi"("Valve Status"=w513, "Station Group"=w512, "Station Number"=w511, "Error In"=w510, "Agilent Valve and Switch Locations"=w506, "Step 3 Input in"=w509, "Day/Night Cycle"=w505, "Semaphore"=w504) -> ("Step 3 Input out"=w508:T6, "Error Out"=w507:errorcluster)  [unwired: 10 in]
    }
    frame 51 {
      n52 = call "WILT Water Valve Control.vi"("Valve Status"=w523, "Station Group"=w522, "Station Number"=w521, "Error In"=w520, "Agilent Valve and Switch Locations"=w516, "Step 3 Input in"=w519, "Day/Night Cycle"=w515, "Semaphore"=w514) -> ("Step 3 Input out"=w518:T6, "Error Out"=w517:errorcluster)  [unwired: 10 in]
    }
    frame 52 {
      n53 = call "WILT Water Valve Control.vi"("Valve Status"=w533, "Station Group"=w532, "Station Number"=w531, "Error In"=w530, "Agilent Valve and Switch Locations"=w526, "Step 3 Input in"=w529, "Day/Night Cycle"=w525, "Semaphore"=w524) -> ("Step 3 Input out"=w528:T6, "Error Out"=w527:errorcluster)  [unwired: 10 in]
    }
    frame 53 {
      n54 = call "WILT Water Valve Control.vi"("Valve Status"=w543, "Station Group"=w542, "Station Number"=w541, "Error In"=w540, "Agilent Valve and Switch Locations"=w536, "Step 3 Input in"=w539, "Day/Night Cycle"=w535, "Semaphore"=w534) -> ("Step 3 Input out"=w538:T6, "Error Out"=w537:errorcluster)  [unwired: 10 in]
    }
    frame 54 {
      n55 = call "WILT Water Valve Control.vi"("Valve Status"=w552, "Station Group"=w553, "Station Number"=w551, "Error In"=w550, "Agilent Valve and Switch Locations"=w546, "Step 3 Input in"=w549, "Day/Night Cycle"=w545, "Semaphore"=w544) -> ("Step 3 Input out"=w548:T6, "Error Out"=w547:errorcluster)  [unwired: 10 in]
    }
    frame 55 {
      n56 = call "WILT Water Valve Control.vi"("Valve Status"=w563, "Station Group"=w562, "Station Number"=w561, "Error In"=w560, "Agilent Valve and Switch Locations"=w556, "Step 3 Input in"=w559, "Day/Night Cycle"=w555, "Semaphore"=w554) -> ("Step 3 Input out"=w558:T6, "Error Out"=w557:errorcluster)  [unwired: 10 in]
    }
    frame 56 {
      n57 = call "WILT Water Valve Control.vi"("Valve Status"=w569, "Station Group"=w573, "Station Number"=w572, "Error In"=w568, "Agilent Valve and Switch Locations"=w566, "Step 3 Input in"=w571, "Day/Night Cycle"=w565, "Semaphore"=w564) -> ("Step 3 Input out"=w570:T6, "Error Out"=w567:errorcluster)  [unwired: 10 in]
    }
  }
  "Error Out" <- w6
  "Step 3 Output" <- w7
  n58 = case shown="\"Turn Valve OFF (Injection 2)\"" "Valve Status" {
    tunnel: [w574 w575 w576 w577] -> w9
    frame "Turn Valve ON (Injection 1)", Default {
      n59 = global read "WILT Globals Main Program.vi" "Run"() -> (w574:u32)
    }
    frame "Turn Valve OFF (Injection 1)" {
      n60 = global read "WILT Globals Main Program.vi" "Watering"() -> (w575:u32)
    }
    frame "Turn Valve ON (Injection 2)" {
      n61 = global read "WILT Globals Main Program.vi" "Watering 2"() -> (w576:u32)
    }
    frame "Turn Valve OFF (Injection 2)" {
      n62 = global read "WILT Globals Main Program.vi" "Watering"() -> (w577:u32)
    }
  }
  n63 = Bundle By Name(cluster="Dryer Step 4 In", "Status Color"=w9) -> (→"Dryer Step 4 Output":T8)
